vi "FP_QTMTelegram_Unpack.vi"(9 "Component\nSize":i32[](array[numeric])=[0, 3, 4, 1, 9, 12, 6, 4, 4, 4, 5, 13, 7], 11 "6DOF telegram":string) -> (1 "FrameNumber":i32, 3 "Data Frame":T1={"Timestamp"=115, "Framenumber"=28, "ComponentCount"=1, "Components"=[{"ComponentSize"=0, "ComponentType"=1, "Count"=0, "Padding"=0, "Data"=[[0.0], [0.0], [0.0], [0.0], [0.0], [0.0]]}]} {"Components"."ComponentType" items=["3D"=1, "3DRes"=9, "3DnoLabels"=2, "Analog"=3, "3DnoLabelsRes"=10, "Force"=4, "6D"=5, "6DRes"=11, "6DEuler"=6, "6DEulerRes"=12, "2D"=7, "2DLin"=8]})   [LabVIEW 2014, in "Oqus Custom Device.lvlib"]
uses:
  Oqus Custom Device.lvlib
  QTM Data Frame.ctl
  QTM ComonentType.ctl
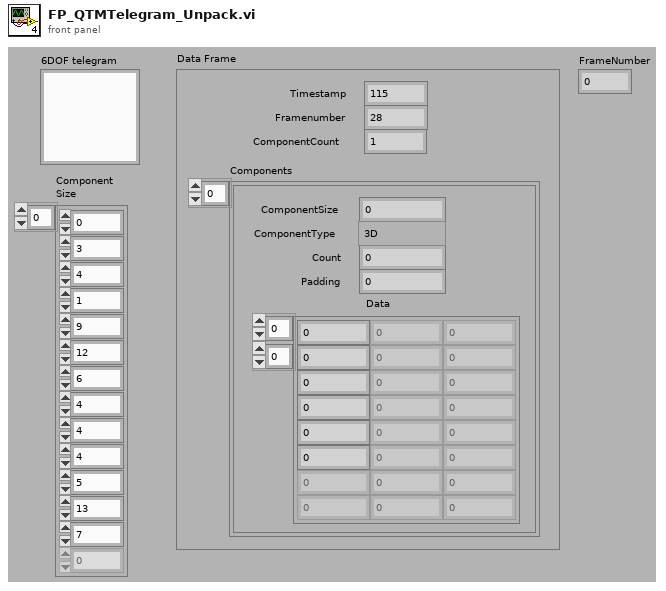
[diagram p1: front panel]
types:
  T1 = typedef "Oqus Custom Device.lvlib/QTM Data Frame.ctl" = cluster{"Timestamp":i64, "Framenumber":i32, "ComponentCount":i32, "Components":cluster{"ComponentSize":i32, "ComponentType":T2, "Count":i32, "Padding":i32, "Data":dbl[][]}[]}
  T2 = typedef "Oqus Custom Device.lvlib/QTM ComonentType.ctl" = i32
  T3 = cluster{"ComponentSize":i32, "ComponentType":T2, "Count":i32, "Padding":i32, "Data":dbl[][]}[]
  T4 = cluster{"ComponentSize":i32, "ComponentType":T2, "Count":i32, "Padding":i32, "Data":dbl[][]}
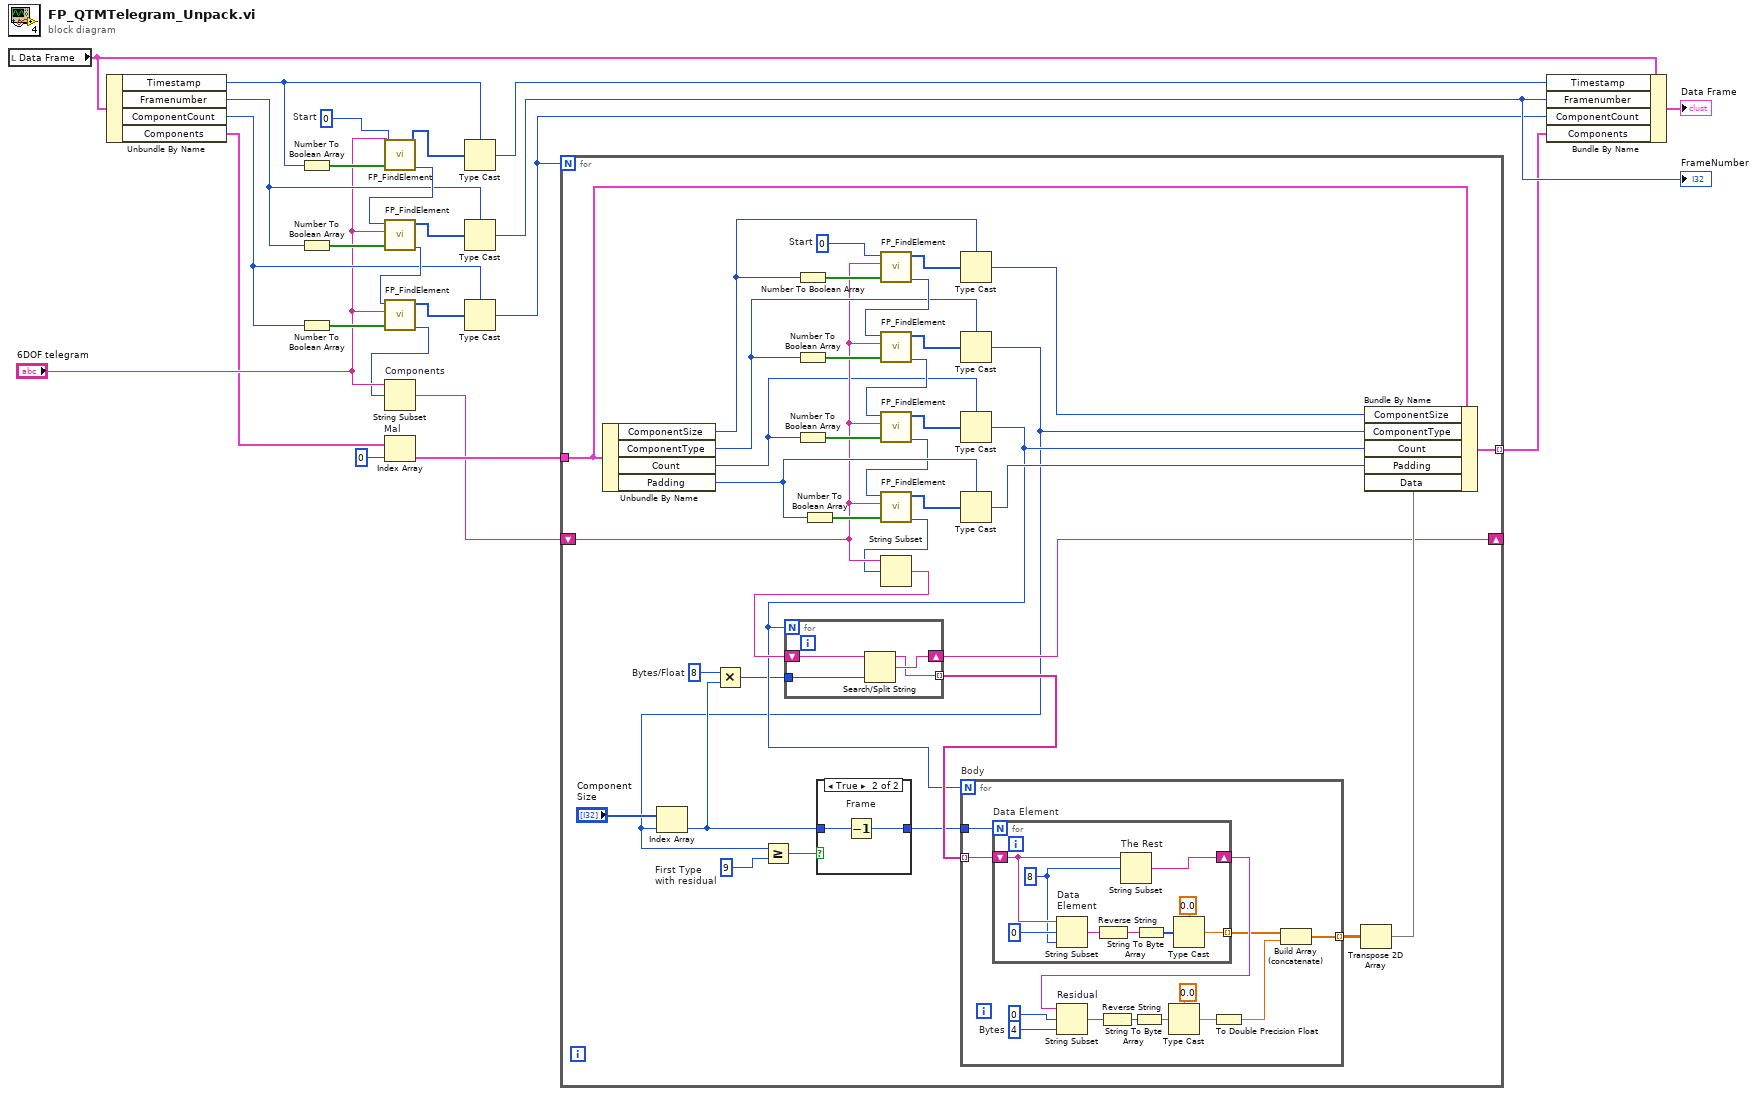
[diagram p0: block diagram]
diagram:
  w23 = 0  # Start
  n1 = local read "Data Frame"() -> (w24:T1)
  n2 = Unbundle By Name(w24) -> ("Timestamp"=w22:i64, "Framenumber"=w15:i32, "ComponentCount"=w11:i32, "Components"=w4:T3)
  n3 = Number To Boolean Array(number=w22) -> (Boolean array=w21:bool[])
  n4 = Number To Boolean Array(number=w15) -> (Boolean array=w18:bool[])
  n5 = Number To Boolean Array(number=w11) -> (Boolean array=w14:bool[])
  n6 = call "FP_FindElement.vi"("Size as Array"=w21, "6DOF telegram"="6DOF telegram", "Start position"=w23) -> ("End position + 1"=w16:i32, "Value"=w20:u8[])  [unwired: 7 out]
  n7 = call "FP_FindElement.vi"("Size as Array"=w18, "6DOF telegram"="6DOF telegram", "Start position"=w16) -> ("End position + 1"=w13:i32, "Value"=w17:u8[])  [unwired: 7 out]
  n8 = call "FP_FindElement.vi"("Size as Array"=w14, "6DOF telegram"="6DOF telegram", "Start position"=w13) -> ("End position + 1"=w7:i32, "Value"=w12:u8[])  [unwired: 7 out]
  n9 = String Subset "Components"(string="6DOF telegram", offset (0)=w7) -> (substring=w1:string)  [unwired: 1 out]
  n10 = Index Array "Mal"(array=w4, index=0) -> (element=w3:T4)
  n11 = Type Cast(type=w22, x=w20) -> (*(type *) &x=w19:i64)
  n12 = Type Cast(type=w15, x=w17) -> (*(type *) &x=w10:i32)
  "FrameNumber" <- w10
  n13 = Type Cast(type=w11, x=w12) -> (*(type *) &x=w9:i32)
  n14 = for {
    N: w9 -> [_]
    shift-right: [w33] -> _
    shift-left: w1 -> [w40]
    tunnel: w3 -> [w46]
    tunnel: [w43] -> w6 mode=indexing
    w25 = 9  # First Type with residual
    w30 = 8  # Bytes/Float
    w52 = 0  # Start
    n15 = Unbundle By Name(w46) -> ("ComponentSize"=w41:i32, "ComponentType"=w51:T2, "Count"=w36:i32, "Padding"=w48:i32)
    n16 = Number To Boolean Array(number=w41) -> (Boolean array=w60:bool[])
    n17 = Number To Boolean Array(number=w51) -> (Boolean array=w58:bool[])
    n18 = Number To Boolean Array(number=w36) -> (Boolean array=w55:bool[])
    n19 = Number To Boolean Array(number=w48) -> (Boolean array=w49:bool[])
    n20 = call "FP_FindElement.vi"("Size as Array"=w60, "6DOF telegram"=w40, "Start position"=w52) -> ("End position + 1"=w56:i32, "Value"=w59:u8[])  [unwired: 7 out]
    n21 = call "FP_FindElement.vi"("Size as Array"=w58, "6DOF telegram"=w40, "Start position"=w56) -> ("End position + 1"=w54:i32, "Value"=w57:u8[])  [unwired: 7 out]
    n22 = call "FP_FindElement.vi"("Size as Array"=w55, "6DOF telegram"=w40, "Start position"=w54) -> ("End position + 1"=w47:i32, "Value"=w53:u8[])  [unwired: 7 out]
    n23 = call "FP_FindElement.vi"("Size as Array"=w49, "6DOF telegram"=w40, "Start position"=w47) -> ("End position + 1"=w37:i32, "Value"=w50:u8[])  [unwired: 7 out]
    n24 = String Subset(string=w40, offset (0)=w37) -> (substring=w35:string)  [unwired: 1 out]
    n25 = Type Cast(type=w41, x=w59) -> (*(type *) &x=w45:i32)
    n26 = Type Cast(type=w51, x=w57) -> (*(type *) &x=w26:T2)
    n27 = Index Array(array="Component\nSize", index=w26) -> (element=w29:i32)
    n28 = Multiply(x=w30, y=w29) -> (x*y=w31:i32)
    n29 = Greater Or Equal?(x=w26, y=w25) -> (x >= y?=w27:bool)
    n30 = case shown="True" w27 {
      tunnel: w29 -> [w61 w63]
      tunnel: [w61 w62] -> w28
      frame False {
      }
      frame True {
        n31 = Decrement "Frame"(x=w63) -> (x-1=w62:i32)
      }
    }
    n32 = Type Cast(type=w36, x=w53) -> (*(type *) &x=w32:i32)
    n33 = for {
      N: w32 -> [_]
      shift-right: [w66] -> w33
      shift-left: w35 -> [w67]
      tunnel: [w65] -> w34 mode=indexing
      tunnel: w31 -> [w64]
      n34 = Search/Split String(string=w67, offset (0)=w64) -> (substring before match=w65:string, match + rest of string=w66:string)  [unwired: 2 out]
    }
    n35 = Type Cast(type=w48, x=w50) -> (*(type *) &x=w44:i32)
    n36 = for "Body" {
      N: w32 -> [_]
      tunnel: w28 -> [w80]
      tunnel: [w74] -> w39 mode=indexing
      tunnel: w34 -> [w79] mode=indexing
      w77 = 4  # Bytes
      n37 = for "Data Element" {
        N: w80 -> [_]
        shift-right: [w84] -> w78
        shift-left: w79 -> [w85]
        tunnel: [w83] -> w73 mode=indexing
        w81 = 8 ("length (rest)")
        n38 = String Subset "Data\nElement"(string=w85, offset (0)=0 ("length (rest)"), length (rest)=w81) -> (substring=w87:string)
        n39 = Reverse String(1:w87) -> (0:w86:string)
        n40 = String Subset "The Rest"(string=w85, offset (0)=w81) -> (substring=w84:string)  [unwired: 1 out]
        n41 = String To Byte Array(string=w86) -> (unsigned byte array=w89:u8[])
        n42 = Type Cast(type=0.0, x=w89) -> (*(type *) &x=w83:dbl)
      }
      n43 = String Subset "Residual"(string=w78, offset (0)=0, length (rest)=w77) -> (substring=w72:string)
      n44 = Reverse String(1:w72) -> (0:w71:string)
      n45 = String To Byte Array(string=w71) -> (unsigned byte array=w75:u8[])
      n46 = Type Cast(type=sgl 0.0, x=w75) -> (*(type *) &x=w69:sgl)
      n47 = To Double Precision Float(number=w69) -> (double precision float=w68:dbl)
      n48 = Build Array (concatenate)(w73, w68) -> (w74:dbl[])
    }
    n49 = Transpose 2D Array(2D array=w39) -> (transposed array=w38:dbl[][])
    n50 = Bundle By Name(cluster=w46, "ComponentSize"=w45, "ComponentType"=w26, "Count"=w32, "Padding"=w44, "Data"=w38) -> (w43:T4)
  }
  n51 = Bundle By Name(cluster=w24, "Timestamp"=w19, "Framenumber"=w10, "ComponentCount"=w9, "Components"=w6) -> (→"Data Frame":T1)
